vi "Read 1 Key Tap Position.vi"(8 "Error In":errorcluster, 11 "Leap Handle":T2) -> (0 "Error Out":errorcluster, 1 "Key Tap Status":T1, 2 "Key Tap Position":cluster{"X":sgl, "Y":sgl, "Z":sgl}, 3 "Leap Handle":T2)   [LabVIEW 2014, in "LMH-Leap.lvlib"]
doc: "Read one key tap gesture position."
uses:
  LMH-Leap.lvlib
  Private/Type Defs/Leap Handle.ctl
  C:/github/makerhub/Leap/LabVIEW/vi.lib/LabVIEW Hacker/Leap/Private/Libs/LeapCSharp.NET3.5.dll
  LabVIEW Hacker/Leap/Private/Libs/LeapCSharp.NET3.5.dll
  Private/Type Defs/Gesture State.ctl
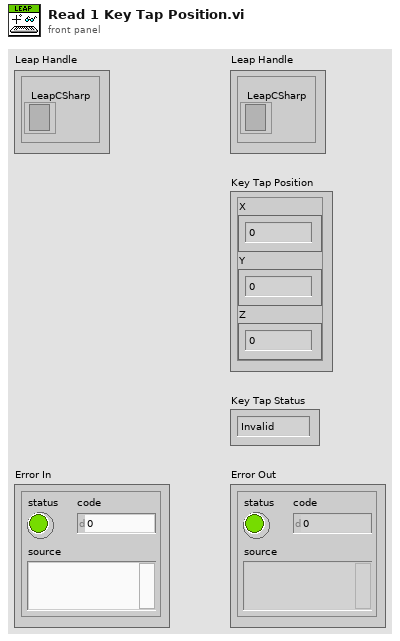
[diagram p1: front panel]
types:
  T1 = typedef "LMH-Leap.lvlib/Gesture State.ctl" = enum16{"Invalid", "Start", "Update", "Stop"}
  T2 = typedef "LMH-Leap.lvlib/Leap Handle.ctl" = cluster{"LeapCSharp":refnum<k24>}
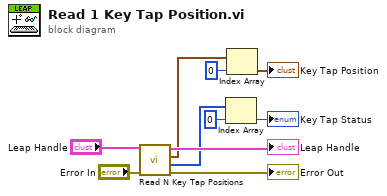
[diagram p0: block diagram]
diagram:
  n1 = call "Read N Key Tap Positions.vi"("Error In"="Error In", "Leap Handle"="Leap Handle") -> ("Error Out"=→"Error Out":errorcluster, "Key Tap Statuses"=w3:T1[], "Key Tap Positions"=w4:cluster{"X":sgl, "Y":sgl, "Z":sgl}[], "Leap Handle"=→"Leap Handle":T2)  [unwired: 6 in]
  n2 = Index Array(array=w3, index=0) -> (element=→"Key Tap Status":T1)
  n3 = Index Array(array=w4, index=0) -> (element=→"Key Tap Position":cluster{"X":sgl, "Y":sgl, "Z":sgl})
